vi "Get Local Chassis Name.vi"(8 "error in":errorcluster, 11 "chassis ref in":T1 format="%.0x") -> (0 "error out":errorcluster, 2 "name":string, 3 "chassis ref out":T1 format="%.0x")   [LabVIEW 2020, in "Scan Engine Scripting.lvlib"]
doc: "Returns the local chassis name from the provided chassis reference."
uses:
  Scan Engine Scripting.lvlib
  <vilib>/NI VeriStand/Custom Device API/Custom Device Item Ref.ctl
  <vilib>/NI VeriStand/Custom Device API/Custom Device API.lvlib
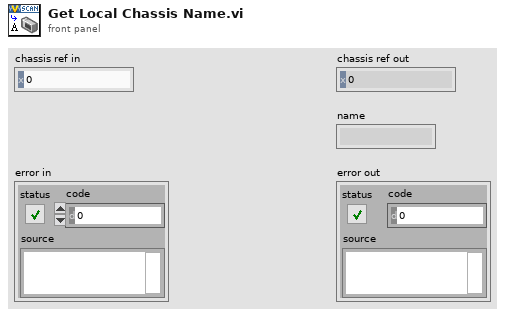
[diagram p1: front panel]
types:
  T1 = typedef "Custom Device API.lvlib/Custom Device Item Ref.ctl" = u64
  T2 = typedef "Custom Device API.lvlib/Custom Device Item Info.ctl" = cluster{"Name":string, "Is Channel":bool, "GUID":string, "Is Waveform":bool}
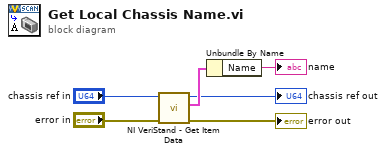
[diagram p0: block diagram]
diagram:
  n1 = call <vilib>:"NI VeriStand - Get Item Data.vi"("error in (no error)"="error in", "Item Ref in"="chassis ref in") -> ("error out"=→"error out":errorcluster, "Item Info"=w2:T2, "Item Ref out"=→"chassis ref out":T1)  [unwired: 7 out]
  n2 = Unbundle By Name(w2) -> ("Name"=→"name":string)
